vi "Select Cluster.vi"(8 "error in (no error)":errorcluster, 11 "Editor in":refnum<class "Editor.lvclass">) -> (0 "error out":errorcluster, 3 "Editor out":refnum<class "Editor.lvclass">)   [LabVIEW 2020, in "VolatusGUIEditor.lvlib" / "Editor.lvclass"]
uses:
  Editor.lvclass
  Editor.lvclass/Editor.ctl
  lv-volatus/VolatusConfig/VolatusConfig/VolatusConfig.lvclass
  lv-volatus/VolatusConfig/VolatusConfig.lvlib
  lv-volatus/VolatusConfig/Meta Type.ctl
  lv-cdm/CDM-Config/Config Element/Config Element.lvclass
panel:
  in  "Cancel":bool
  in  "Select":bool
  in  "Listbox":i32(listbox)
  # "Multiple clusters are available for this system, please select the cluster the GUI is a part of:"
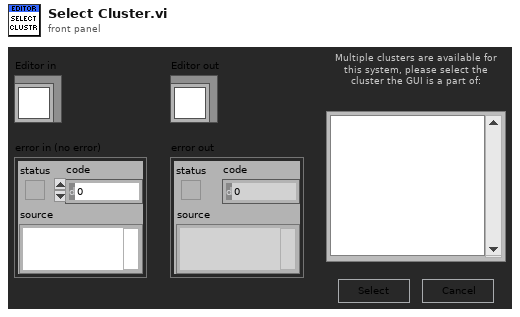
[diagram p1: front panel]
types:
  T1 = typedef "VolatusConfig.lvlib/Meta Type.ctl" = enum16{"UNKNOWN", "VL_System", "VL_Cluster", "VL_Node", "VL_Task", "VL_Group", "VL_Channel", "VL_Task_List", "VL_Scaling", "VL_Sensor", "VL_Sensor_List", "VL_Scale"}
  T2 = enum32{"Invalid", "Standard", "Closed", "Hidden", "Minimized", "Maximized"}
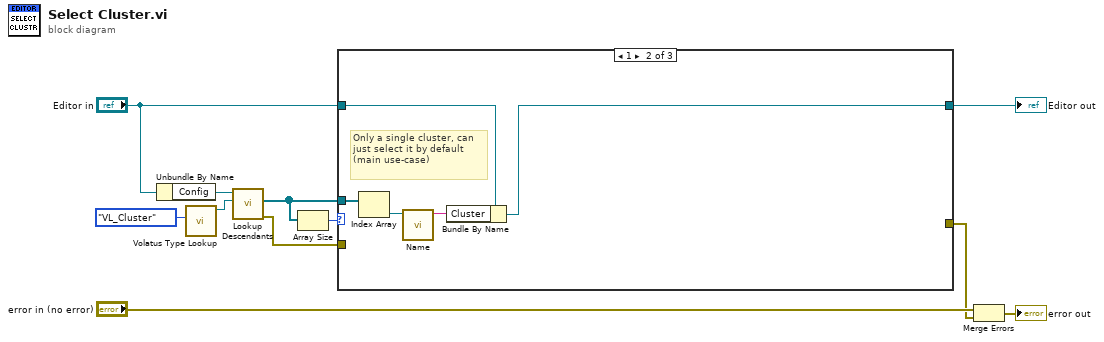
[diagram p0: block diagram]
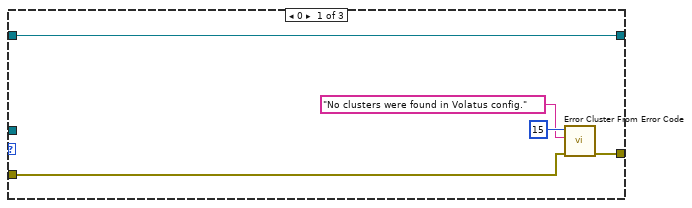
[diagram p2: hidden frame]
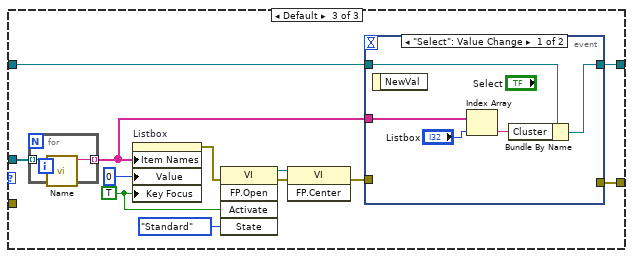
[diagram p3: hidden frame]
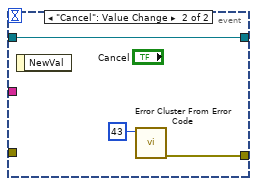
[diagram p4: hidden frame]
diagram:
  n1 = Unbundle By Name("Editor in") -> ("Config"=w10:refnum<class "VolatusConfig.lvclass">)
  n2 = call "Volatus Type Lookup.vi"("Meta Type"=Meta_Type."VL_Cluster") -> ("Config Lookup out"=w8:refnum<class "Config Lookup.lvclass">)  [unwired: 9 in, 1 out]
  n3 = call "Lookup Descendants.vi"("Lookup"=w8, "VolatusConfig in"=w10) -> ("error out"=w3:errorcluster, "Descendants"=w4:refnum<class "Config Element.lvclass">[])  [unwired: 7 in, 1 out]
  n4 = Array Size(array=w4) -> (size(s)=w7:i32)
  n5 = case shown="1" w7 {
    tunnel: "Editor in" -> [w16 w19 w31]
    tunnel: [w16 w17 w29] -> w5
    tunnel: w4 -> [_ w21 w33]
    tunnel: [w15 _ w28] -> w1
    tunnel: w3 -> [w12 _ _]
    frame 0 {
      n6 = call <vilib>:"Error Cluster From Error Code.vi"("error in (no error)"=w12, "error message (\"\")"="No clusters were found in Volatus config.", "error code (0)"=15) -> ("error out"=w15:errorcluster)  [unwired: 6 in]
    }
    frame 1 {
      # "Only a single cluster, can just select it by default (main use-case)"
      n7 = Index Array(array=w21) -> (element=w20:refnum<class "Config Element.lvclass">)  [unwired: 1 in]
      n8 = call "Name.vi"("Config Element in"=w20) -> ("Name"=w18:string)  [unwired: 9 in, 1 out]
      n9 = Bundle By Name(cluster=w19, "Cluster"=w18) -> (w17:refnum<class "Editor.lvclass">)
    }
    frame Default {
      w26 = TRUE ("Key Focus")
      n10 = for {
        tunnel: w33 -> [w35] mode=indexing
        tunnel: [w34] -> w30 mode=indexing
        n11 = call "Name.vi"("Config Element in"=w35) -> ("Name"=w34:string)  [unwired: 9 in, 1 out]
      }
      n12 = property on="Listbox" class="LstBox (strict)"("Item Names"=w30, "Value"=0 ("Listbox"), "Key Focus"=w26) -> (error out=w27:errorcluster)  [unwired: 2 in, 1 out]
      n13 = invoke class="VI" method="FP.Open"(error in=w27, "Activate"=w26, "State"=T2."Standard") -> (reference out=w24:refnum<vi>, error out=w23:errorcluster)  [unwired: 2 in, 3 out]
      n14 = invoke class="VI" method="FP.Center"(reference=w24, error in=w23) -> (error out=w22:errorcluster)  [unwired: 1 in, 2 out]
      n15 = event shown="[0] \"Select\": Value Change" {
        selector: _ -> [_ _]
        dyn-events: _ -> [_ _]
        timeout: _ -> [_ _]
        tunnel: w31 -> [w38 w43]
        tunnel: w30 -> [w40 _]
        tunnel: [w36 w43] -> w29
        tunnel: [_ w41] -> w28
        tunnel: w22 -> [_ _]
        event "Select": Value Change {
          n16 = event-data() -> ()  [unwired: 1 in, 1 out]
          n17 = Index Array(array=w40, index="Listbox") -> (element=w37:string)
          n18 = Bundle By Name(cluster=w38, "Cluster"=w37) -> (w36:refnum<class "Editor.lvclass">)
        }
        event "Cancel": Value Change {
          n19 = event-data() -> ()  [unwired: 1 in, 1 out]
          n20 = call <vilib>:"Error Cluster From Error Code.vi"("error code (0)"=43) -> ("error out"=w41:errorcluster)  [unwired: 8 in]
        }
      }
    }
  }
  "Editor out" <- w5
  n21 = Merge Errors("error in (no error)", w1) -> (→"error out":errorcluster)
